vi "Fishing Continuous OCR wit Max Likelihood.vi"() -> ()   [LabVIEW 2019]
doc: "This VI captures the region of the screen and displays it on the front panel continuously.\nCan be used to develop remote desktop applications."
uses:
  <vilib>/Utility/miscctls.llb/LVBoundsTypeDef.ctl
  System.Drawing
  <vilib>/Instr/_visa.llb/VISA Configure Serial Port (Instr).vi
  <vilib>/Utility/inputDevices.llb/mouseAcquire.vi
  <vilib>/Utility/inputDevices.llb/closeMouse.vi
  <vilib>/wsapi/NI_WebServices.lvlib
panel:
  out "Buffer Reset":bool
  out "Array Reset":bool
  out "TXB":bool
  out "Scan Cycle":dbl
  out "read buffer":string
  out "Max Likelihood Output":string
  out "Max Index":i32
  in  "Manual Reset Array":bool
  out "Input Likelihood":dbl[](array[numeric])
  out "Possible Inputs":string[](array[string])
  out "Init Error":errorcluster
  out "Length":i32
  out "Tx":string
  in  "String Cont":string
  out "Return Count":u32
  out "COM Status":bool
  in  "MC COM Port":refnum<visa-resource-name>="COM5"
  out "Processed Image":T1(plugin-control)
  out "Filtered String Output":string
  in  "Delay (ms)":i32=100
  in  "Error In":errorcluster
  out "Mouse y":dbl
  out "Mouse x":dbl
  in  "Height (px)":i32=100
  in  "Width (px)":i32=600
  out "Screen Capture":picture
  in  "stop":bool
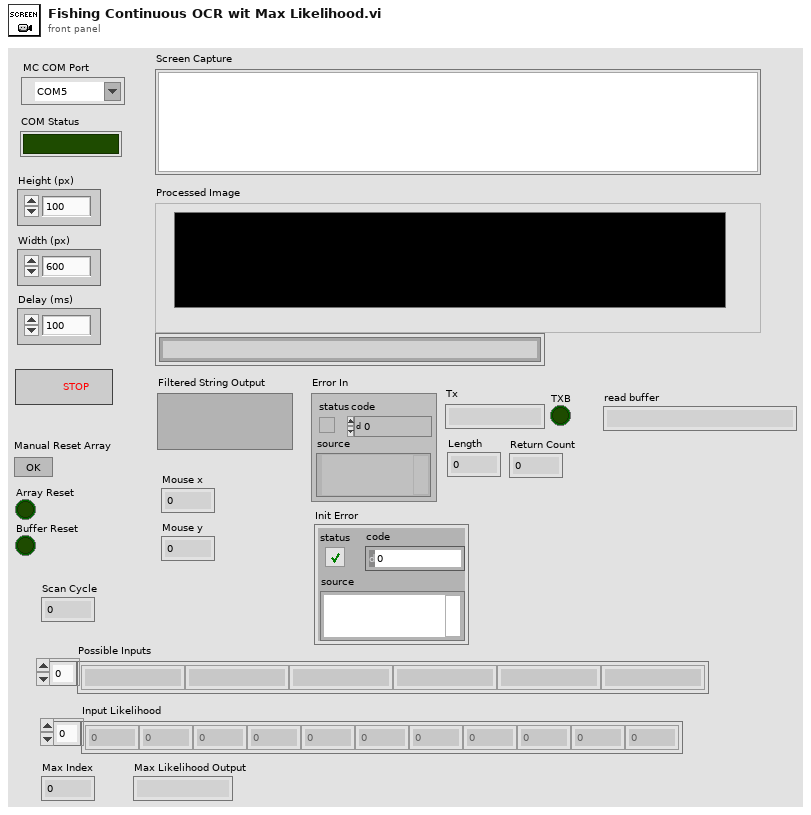
[diagram p1: front panel]
types:
  T1 = typedef "IMAQ Image.ctl" = refnum<image>
  T2 = typedef "LVBoundsTypeDef.ctl" = cluster{"Width":u32, "Height":u32}
  T3 = typedef "Image Type" = u32
  T4 = cluster{"Horizontal":i32, "Vertical":i32, "Scrolling":i32}
  T5 = typedef "imagedata.ctl" = cluster{"image type":i32, "image depth":i32, "image":u8[], "mask":u8[], "colors":u32[], "Rectangle":cluster{"left":i16, "top":i16, "right":i16, "bottom":i16}}
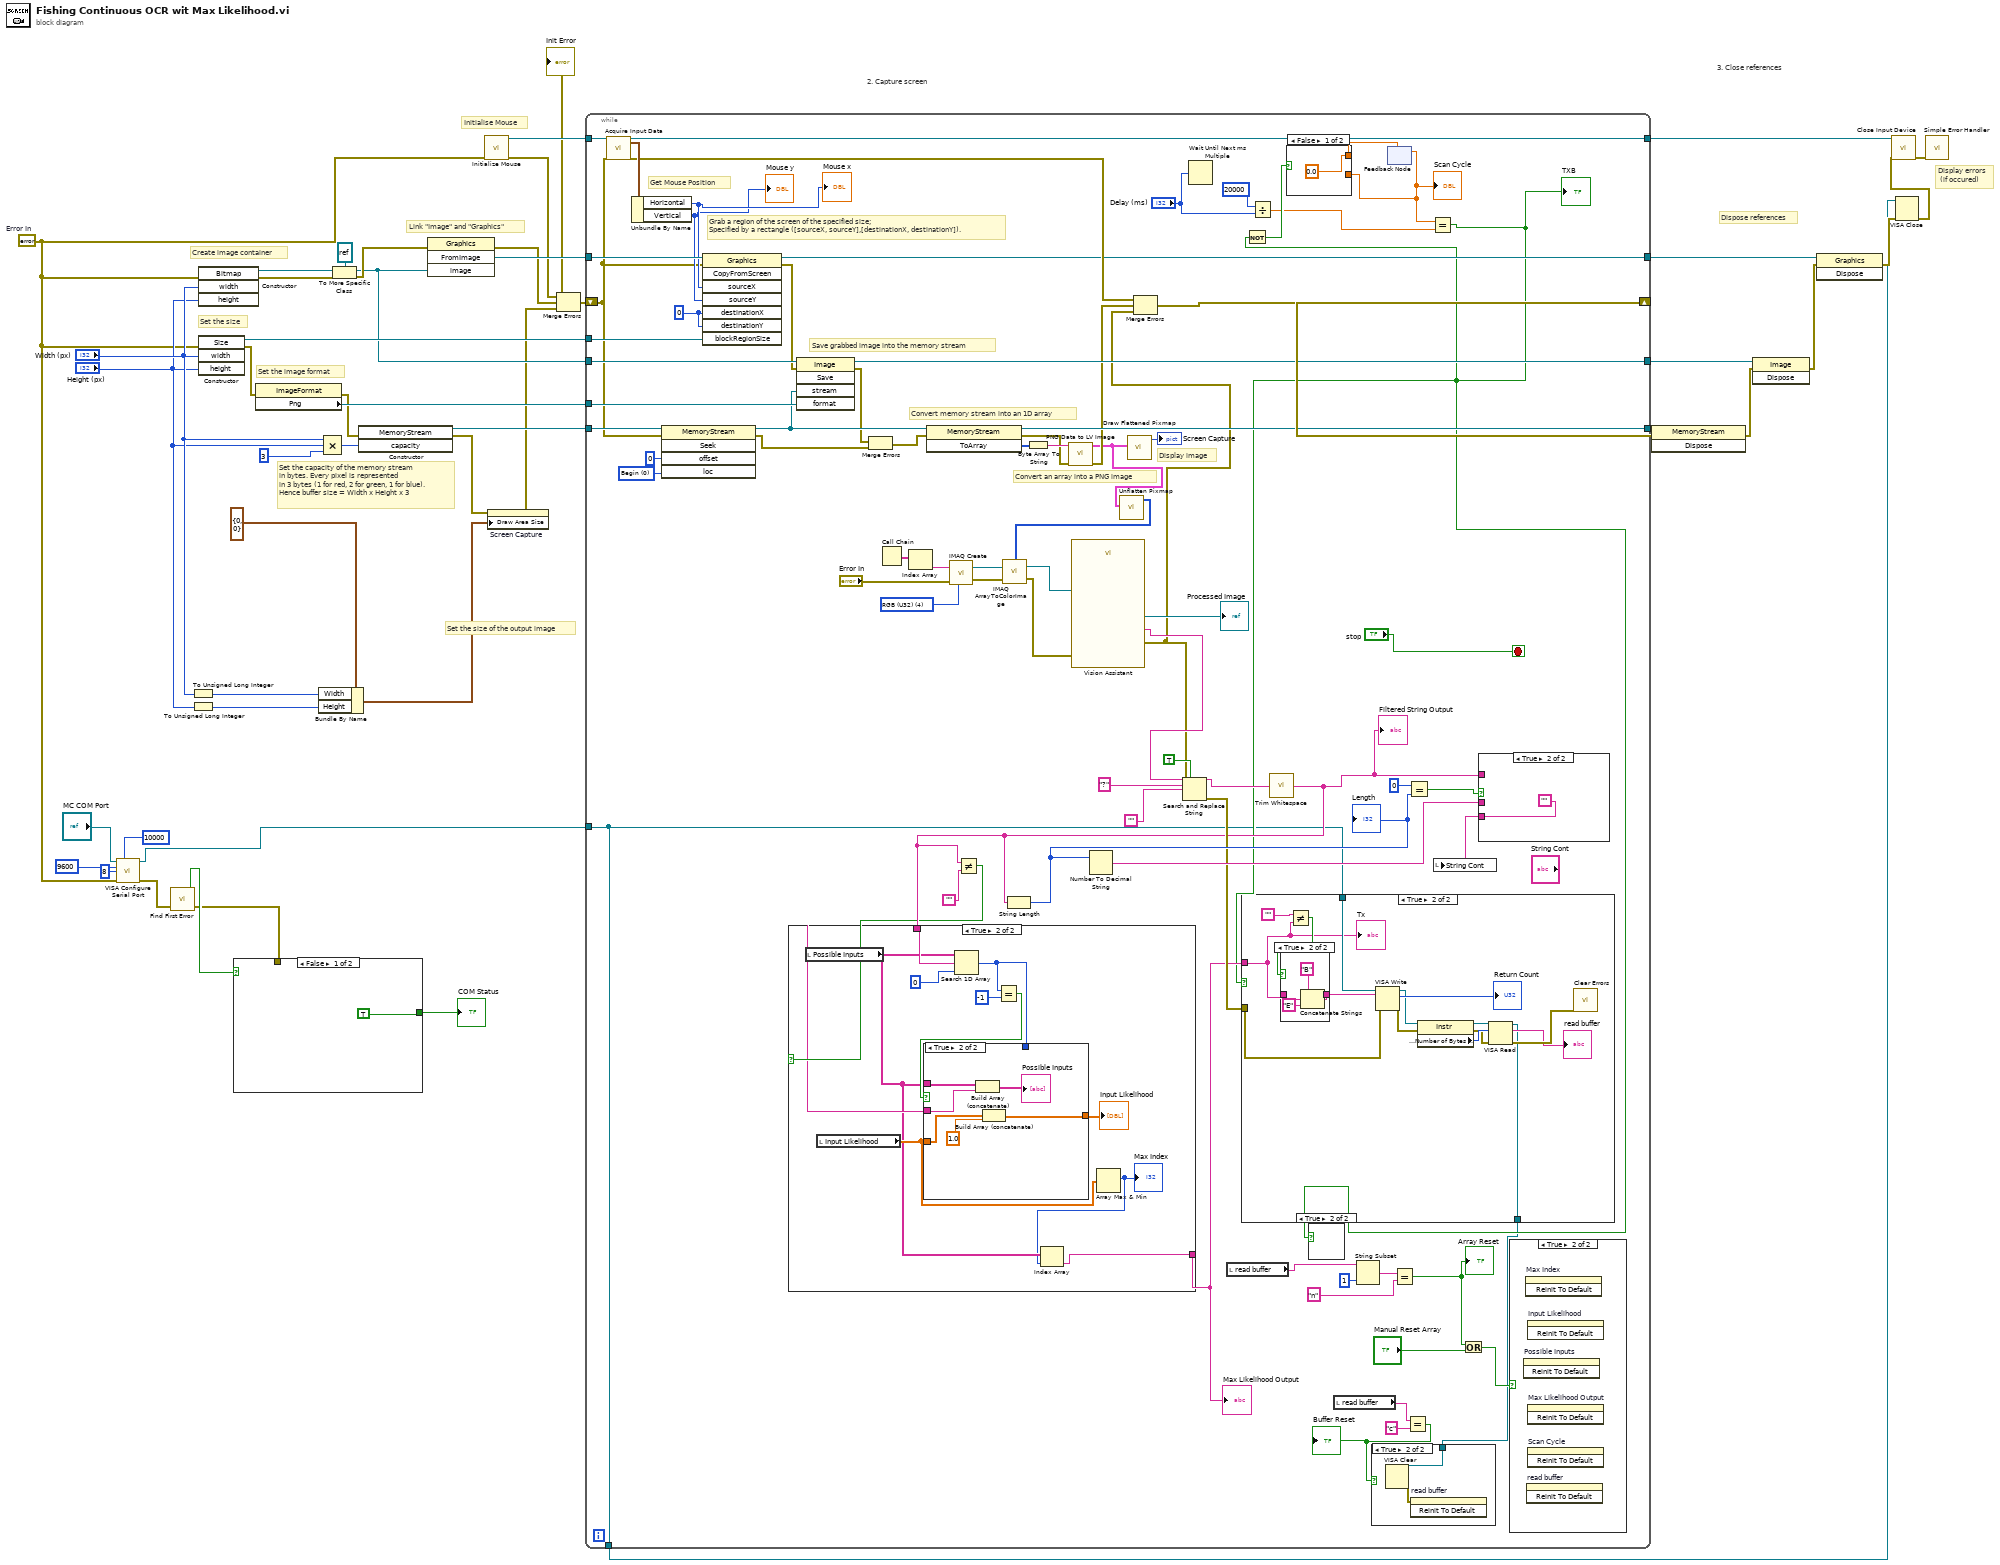
[diagram p0: block diagram]
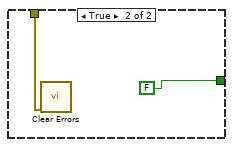
[diagram p2: hidden frame]
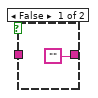
[diagram p6: hidden frame]
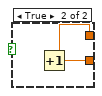
[diagram p7: hidden frame]
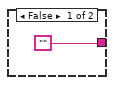
[diagram p8: hidden frame]
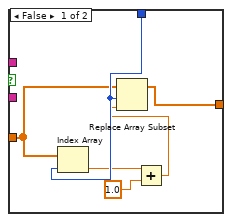
[diagram p9: hidden frame]
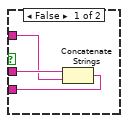
[diagram p11: hidden frame]
diagram:
  w12 = errorcluster {"status"=FALSE, "code"=0, "source"=""}  # Error In
  # "Link \"Image\" and \"Graphics\""
  # "Set the size"
  # "Create image container"
  # "3. Close references"
  # "2. Capture screen"
  # "Display errors\n (if occured)"
  # "Dispose references"
  # "Set the image format"
  # "Set the size of the output image"
  # "Set the capacity of the memory stream\nin bytes. Every pixel is represented\nin 3 bytes (1 for red, 2 for green, 1 for blue).\nHence buffer size = Width x Height x 3"
  # "Initialise Mouse"
  n1 = call-poly "VISA Configure Serial Port"("VISA resource name"="MC COM Port", "timeout (10sec)"=u32 10000, "baud rate (9600)"=u32 9600, "data bits (8)"=u16 8, "error in (no error)"=w12) -> ("VISA resource name out"=w1:refnum<visa-resource-name>, "error out"=w11:errorcluster)  [unwired: 9 in]
  n2 = call <vilib>:"Find First Error.vi"("error in (no error)"=w11) -> ("error out"=w8:errorcluster, "error?"=w10:bool)  [unwired: 3 in]
  n3 = To Unsigned Long Integer(number="Width (px)") -> (unsigned 32bit integer=w20:u32)
  n4 = To Unsigned Long Integer(number="Height (px)") -> (unsigned 32bit integer=w18:u32)
  n5 = constructor class="Bitmap"(error in=w12, "width"="Width (px)", "height"="Height (px)") -> (reference out=w40:refnum<k24>, error out=w43:errorcluster)  [unwired: 2 in, 3 out]
  n6 = constructor class="Size"(error in=w12, "width"="Width (px)", "height"="Height (px)") -> (reference out=w38:refnum<k24>, error out=w29:errorcluster)  [unwired: 2 in, 3 out]
  n7 = case shown="False" w10 {
    tunnel: [TRUE FALSE] -> w9
    tunnel: w8 -> [_ w48]
    frame False {
    }
    frame True {
      n8 = call <vilib>:"Clear Errors.vi"("error in (no error)"=w48) -> ()  [unwired: 5 in, 2 out]
    }
  }
  "COM Status" <- w9
  n9 = property class="ImageFormat"(error in=w29) -> (error out=w28:errorcluster, "Png"=w37:refnum<k24>)  [unwired: 1 in, 1 out]
  n10 = Bundle By Name(cluster=T2 {"Width"=0, "Height"=0} ("Draw Area Size"), "Width"=w20, "Height"=w18) -> (w24:T2)
  n11 = Compound Arithmetic op=MULTIPLY("Width (px)", "Height (px)", 3 ("value")) -> (w32:i32)
  n12 = To More Specific Class(target class=refnum<k24> refnum, reference=w40, error in=w43) -> (specific class reference=w31:refnum<k24>, error out=w44:errorcluster)
  n13 = constructor class="MemoryStream"(error in=w28, "capacity"=w32) -> (reference out=w34:refnum<k24>, error out=w23:errorcluster)  [unwired: 2 in, 2 out]
  n14 = invoke class="Graphics" method="FromImage"(error in=w44, "image"=w31) -> (error out=w27:errorcluster, "FromImage"=w41:refnum<k24>)  [unwired: 2 in, 2 out]
  n15 = call <vilib>:"Initialize Mouse.vi"("error in (no error)"=w12) -> ("error out"=w25:errorcluster, "device ID"=w46:refnum<k1>)  [unwired: 9 in]
  n16 = property on="Screen Capture" class="Pict"(error in=w23, "Draw Area Size"=w24) -> (error out=w22:errorcluster)  [unwired: 1 in, 1 out]
  n17 = Merge Errors(w25, w27, w22) -> (w26:errorcluster)
  "Init Error" <- w26
  n18 = while {
    tunnel: w46 -> [w125]
    tunnel: [w123] -> w45
    tunnel: w41 -> [w122]
    tunnel: [w119] -> w39
    tunnel: w38 -> [w118]
    tunnel: w37 -> [w117]
    tunnel: [w116] -> w36
    tunnel: w34 -> [w115]
    tunnel: w31 -> [w109]
    shift-right: [w101] -> w14
    shift-left: w26 -> [w80]
    tunnel: [w100] -> w17
    tunnel: w1 -> [w54]
    tunnel: [w54] -> w5
    stop <- "stop" stop-if-true
    w92 = T3 4 items=["Grayscale (U8)", "Grayscale (I16)", "Grayscale (SGL)", "Complex (CSG)", "RGB (U32)", "HSL (U32)", "RGB (U64)", "Grayscale (U16)"] ("Image Type")
    w110 = 0 ("destinationX")
    w113 = 0 items=["Begin", "Current", "End"] ("loc")
    # "Display image"
    # "Convert an array into a PNG image"
    # "Convert memory stream into an 1D array"
    # "Save grabbed image into the memory stream"
    # "Grab a region of the screen of the specified size;\nSpecified by a rectangle ([sourceX, sourceY],[destinationX, destinationY])."
    # "Get Mouse Position"
    n19 = call-poly <vilib>:"Acquire Input Data.vi"("device ID"=w125, "error in (no error)"=w80) -> ("device ID"=w123:refnum<k1>, "axis info"=w124:T4, "error out"=w103:errorcluster)  [unwired: 14 in, 1 out]
    n20 = Unbundle By Name(w124) -> ("Horizontal"=w99:i32, "Vertical"=w98:i32)
    "Mouse x" <- w99
    "Mouse y" <- w98
    n21 = invoke class="MemoryStream" method="Seek"(reference=w115, error in=w80, "offset"=i64 0, "loc"=w113) -> (reference out=w111:refnum<k24>, error out=w106:errorcluster)  [unwired: 1 in, 3 out]
    n22 = invoke class="Graphics" method="CopyFromScreen"(reference=w122, error in=w80, "sourceX"=w99, "sourceY"=w98, "destinationX"=w110, "destinationY"=w110, "blockRegionSize"=w118) -> (reference out=w100:refnum<k24>, error out=w104:errorcluster)  [unwired: 1 in, 6 out]
    n23 = invoke class="Image" method="Save"(reference=w109, error in=w104, "stream"=w111, "format"=w117) -> (reference out=w116:refnum<k24>, error out=w107:errorcluster)  [unwired: 1 in, 3 out]
    n24 = Merge Errors(w107, w106) -> (w105:errorcluster)
    n25 = Call Chain() -> (call chain=w94:string[])
    n26 = Index Array(array=w94) -> (element=w95:string)  [unwired: 1 in]
    n27 = invoke class="MemoryStream" method="ToArray"(reference=w111, error in=w105) -> (reference out=w119:refnum<k24>, error out=w108:errorcluster, "ToArray"=w121:u8[])  [unwired: 1 in]
    n28 = call "IMAQ Create"("Image Name"=w95, "Image Type"=w92, "error in (no error)"="Error In") -> ("New Image"=w91:T1, "error out"=w90:errorcluster)  [unwired: 1 in, 1 out]
    n29 = Byte Array To String(unsigned byte array=w121) -> (string=w120:string)
    n30 = call <vilib>:"PNG Data to LV Image.vi"("error in (no error)"=w108, "png data"=w120) -> ("error out"=w102:errorcluster, "image data"=w97:T5)  [unwired: 8 in]
    n31 = call <vilib>:"Unflatten Pixmap.vi"("image data"=w97) -> ("24-bit pixmap"=w96:u32[][])  [unwired: 4 in, 6 out]
    n32 = call "IMAQ ArrayToColorImage"("Image Pixels (U32)"=w96, "Image"=w91, "error in (no error)"=w90) -> ("Image Out"=w88:T1, "error out"=w89:errorcluster)  [unwired: 2 in]
    n33 = call "Vision Assistant"("Image In"=w88, "error in"=w89) -> ("Image Out"=→"Processed Image":T1, "String (OCR/OCV 2)"=w84:string, "error out"=w74:errorcluster)  [unwired: 23 in]
    n34 = call <vilib>:"Draw Flattened Pixmap.vi"("image data"=w97) -> ("new picture"=→"Screen Capture":picture)  [unwired: 8 in]
    n35 = Merge Errors(w103, w102, w74) -> (w101:errorcluster)
    n36 = Search and Replace String(replace all?=TRUE ("replace all? (F)"), input string=w84, search string="?", replace string="", error in=w74) -> (result string=w83:string, error out=w73:errorcluster)  [unwired: 3 in, 2 out]
    n37 = Wait Until Next ms Multiple(millisecond multiple="Delay (ms)") -> ()  [unwired: 1 out]
    n38 = local read "read buffer"() -> (w57:string)
    n39 = Divide(x=20000, y="Delay (ms)") -> (x/y=w61:dbl)
    n40 = call <vilib>:"Trim Whitespace.vi"("string"=w83) -> ("trimmed string"=w71:string)  [unwired: 1 in]
    "Filtered String Output" <- w71
    n41 = Not Equal?(x=w71, y="") -> (x != y?=w70:bool)
    n42 = case shown="True" w70 {
      tunnel: w71 -> [_ w157]
      tunnel: ["" w153] -> w69
      frame False {
      }
      frame True {
        n43 = local read "Possible Inputs"() -> (w155:string[])
        n44 = local read "Input Likelihood"() -> (w156:dbl[])
        n45 = Search 1D Array(1D array=w155, element=w157, start index (0)=0) -> (index of element=w159:i32)
        n46 = Equal?(x=w159, y=-1) -> (x = y?=w160:bool)
        n47 = case shown="True" w160 {
          tunnel: w155 -> [_ w174]
          tunnel: w157 -> [_ w173]
          tunnel: w159 -> [w168 _]
          tunnel: w156 -> [w164 w170]
          tunnel: [w163 w171] -> w158
          frame False {
            n48 = Index Array(array=w164, index=w168) -> (element=w166:dbl)
            n49 = Add(x=w166, y=1.0) -> (x+y=w165:dbl)
            n50 = Replace Array Subset(array=w164, new element=w165, index=w168) -> (w163:dbl[])
          }
          frame True {
            n51 = Build Array (concatenate)(w174, w173) -> (→"Possible Inputs":string[])
            n52 = Build Array (concatenate)(w170, 1.0 ("new element/subarray")) -> (w171:dbl[])
          }
        }
        "Input Likelihood" <- w158
        n53 = Array Max & Min(array=w156) -> (max index (indices)=w154:i32)  [unwired: 3 out]
        "Max Index" <- w154
        n54 = Index Array(array=w155, index=w154) -> (element=w153:string)
      }
    }
    "Max Likelihood Output" <- w69
    n55 = String Length(string=w71) -> (length=w78:i32)
    "Length" <- w78
    n56 = Number To Decimal String(number=w78) -> (decimal integer string=w76:string)  [unwired: 1 in]
    n57 = local read "read buffer"() -> (w53:string)
    n58 = String Subset(string=w57, length (rest)=1 ("length (rest)")) -> (substring=w55:string)  [unwired: 1 in]
    n59 = feedback #1() -> (w63:dbl)  [unwired: 1 in]
    "Scan Cycle" <- w63
    n60 = Equal?(x=w55, y="n") -> (x = y?=w59:bool)
    "Array Reset" <- w59
    n61 = Equal?(x=w53, y="c") -> (x = y?=w52:bool)
    "Buffer Reset" <- w52
    n62 = Equal?(x=0, y=w78) -> (x = y?=w79:bool)
    n63 = Equal?(x=w63, y=w61) -> (x = y?=w58:bool)
    "TXB" <- w58
    n64 = case shown="True" w58 {
      tunnel: w54 -> [w128 w143]
      tunnel: w73 -> [_ w141]
      tunnel: w69 -> [_ w130]
      tunnel: [w128 w129] -> w51
      frame False {
      }
      frame True {
        n65 = Not Equal?(x="", y=w130) -> (x != y?=w132:bool)
        n66 = case shown="True" w132 {
          tunnel: ["" w148] -> w133
          tunnel: w130 -> [_ w147]
          frame False {
          }
          frame True {
            n67 = Concatenate Strings("B" ("string"), w147, "E" ("string")) -> (w148:string)
          }
        }
        n68 = VISA Write(VISA resource name=w143, write buffer=w133, error in (no error)=w141) -> (VISA resource name out=w140:refnum<visa-resource-name>, return count=→"Return Count":u32, error out=w139:errorcluster)
        n69 = property class="Instr"(reference=w140, error in=w139) -> (reference out=w138:refnum<visa-resource-name>, error out=w136:errorcluster, "Serial Settings:Number of Bytes at Serial Port"=w137:u32)
        n70 = VISA Read(VISA resource name=w138, byte count=w137, error in (no error)=w136) -> (VISA resource name out=w129:refnum<visa-resource-name>, read buffer=→"read buffer":string, error out=w135:errorcluster)  [unwired: 1 out]
        n71 = call <vilib>:"Clear Errors.vi"("error in (no error)"=w135) -> ()  [unwired: 5 in, 2 out]
        "Tx" <- w130
      }
    }
    n72 = Not(x=w58) -> (.not. x?=w64:bool)
    n73 = case shown="False" w64 {
      tunnel: [0.0 w151] -> w65
      tunnel: w63 -> [_ w150]
      frame False {
      }
      frame True {
        n74 = Increment(x=w150) -> (x+1=w151:dbl)
      }
    }
    n75 = case shown="True" w58 {
      frame False {
      }
      frame True {
      }
    }
    n76 = case shown="True" w52 {
      tunnel: w51 -> [_ w127]
      frame False {
      }
      frame True {
        n77 = VISA Clear(VISA resource name=w127) -> (error out=w126:errorcluster)  [unwired: 1 in, 1 out]
        n78 = invoke on="read buffer" class="Str" method="Reinit To Default"(error in=w126) -> ()  [unwired: 2 in, 3 out]
      }
    }
    n79 = feedback-in #1(w65) -> ()
    n80 = Or(x=w59, y="Manual Reset Array") -> (x .or. y?=w68:bool)
    n81 = case shown="True" w79 {
      tunnel: w76 -> [w177 _]
      tunnel: w71 -> [w176 _]
      tunnel: [w175 ""] -> w75
      frame False {
        n82 = Concatenate Strings(w177, w176) -> (w175:string)
      }
      frame True {
      }
    }
    n83 = local write "String Cont"(w75) -> ()
    n84 = case shown="True" w68 {
      frame False {
      }
      frame True {
        n85 = invoke on="Possible Inputs" class="Arr (strict)" method="Reinit To Default"() -> ()  [unwired: 3 in, 3 out]
        n86 = invoke on="Max Index" class="DigNum (strict)" method="Reinit To Default"() -> ()  [unwired: 3 in, 3 out]
        n87 = invoke on="read buffer" class="Str" method="Reinit To Default"() -> ()  [unwired: 3 in, 3 out]
        n88 = invoke on="Input Likelihood" class="Arr (strict)" method="Reinit To Default"() -> ()  [unwired: 3 in, 3 out]
        n89 = invoke on="Max Likelihood Output" class="Str" method="Reinit To Default"() -> ()  [unwired: 3 in, 3 out]
        n90 = invoke on="Scan Cycle" class="DigNum (strict)" method="Reinit To Default"() -> ()  [unwired: 3 in, 3 out]
      }
    }
  }
  n91 = invoke class="MemoryStream" method="Dispose"(reference=w39, error in=w14) -> (error out=w35:errorcluster)  [unwired: 1 in, 2 out]
  n92 = invoke class="Image" method="Dispose"(reference=w36, error in=w35) -> (error out=w16:errorcluster)  [unwired: 1 in, 2 out]
  n93 = invoke class="Graphics" method="Dispose"(reference=w17, error in=w16) -> (error out=w7:errorcluster)  [unwired: 1 in, 2 out]
  n94 = VISA Close(VISA resource name=w5, error in (no error)=w7) -> (error out=w6:errorcluster)
  n95 = call-poly <vilib>:"Close Input Device.vi"("error in (no error)"=w6, "device ID"=w45) -> ("error out"=w15:errorcluster)  [unwired: 8 in]
  n96 = call <vilib>:"Simple Error Handler.vi"("error in (no error)"=w15) -> ()  [unwired: 4 in, 5 out]
